vi "Reset.vi"(8 "error in":errorcluster, 11 "SR 3XX HVPS in":refnum<class "SR 3XX HVPS.lvclass">) -> (0 "error out":errorcluster, 3 "SR 3XX HVPS out":refnum<class "SR 3XX HVPS.lvclass">)   [LabVIEW 2014, in "SR 3XX HVPS.lvclass"]
doc: "The *RST common command resets the PS300 to its default configurations. It is the same as holding down \"CLR \" at power on."
uses:
  SR 3XX HVPS.lvclass
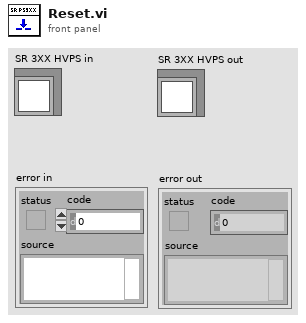
[diagram p1: front panel]
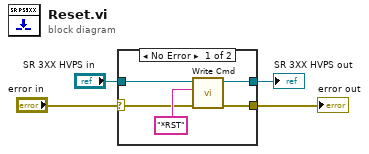
[diagram p0: block diagram]
diagram:
  n1 = case shown="No Error" "error in" {
    selector: "error in" -> [w7 w11]
    tunnel: [w5 w11] -> w3
    tunnel: [w6 w10] -> w1
    tunnel: "SR 3XX HVPS in" -> [w9 w10]
    frame No Error {
      n2 = call "Write Cmd.vi"("error in"=w7, "Cmd"="*RST", "SR 3XX HVPS in"=w9) -> ("error out"=w5:errorcluster, "SR 3XX HVPS out"=w6:refnum<class "SR 3XX HVPS.lvclass">)  [unwired: 7 in]
    }
    frame Error {
    }
  }
  "error out" <- w3
  "SR 3XX HVPS out" <- w1
